vi "GetAlazar_SynthFocus_25.vi"(0 "AlazarCluster":T8, 1 "Digitizer Settings":T4={"Digitizer delay (us) "=0.0, "rf points per line"=2048, "lines per plane"=128, "Samp Rate (Hz)"=100000000.0, "Additional dig delay (us)"=0.0, "Voltage Scale"=0.4, "Pre-Looks"=0, "Offset delay (us)"=0.0, "bits A/D"=8, "Avg Num"=1, "DigTimeOut"=5.0, "Rel Dig Delay"=0.0, "Dig Ch"=0, "LeCroyCluster"={"LeCroy Channels"=[TRUE, FALSE, FALSE, FALSE], "LC read pt offset"=0.0, "Sweep Avg"=FALSE}, "Main Digitizer"=enum."NI Digitizer", "Dig Config"=enum."Single channel", "Digitizer ID Cluster"={"Acqiris/Alazar/SP ID"=[], "NI Instr Handles"=[], "LeCroy VISA"="", "GaGe Handle"={"Handle"=0, "Sample size"=0, "Resolution"=0, "Offset"=0, "Channels"=0, "Boards"=0}, "ATS Ref"="ATS9350", "Acqiris Address"=["PCI::INSTR0"], "ADQRef"=refnum, "adq_cu_ptr"=refnum}, "Trigger Settings"={"Trig Source"=1, "Trig Coupling"=0, "Trig Slope"=0, "Level (mV)"=1500.0}, "Bulk Acq"=FALSE, "Bulk Start Indexes"=[], "Data Ref RF"=refnum, "NI ID/Channel"=[], "Total Dig CH"=1, "Xtra Ann Trig delay (us)"=10.0, "Fix Z Delay?"=FALSE, "One Way Transmission?"=FALSE, "Data Ref Log"=refnum} {"Trigger Settings"."Trig Slope" items=["Positive", "Negative"]; "Trigger Settings"."Level (mV)" format="%.2f"; "Trigger Settings"."Trig Coupling" items=["DC 1 MOhm", "AC 1 MOhm", "DC 50 Ohm", "AC 50 Ohm"]; "Trigger Settings"."Trig Source" items=["Chan 1", "External"]; "Rel Dig Delay" format="%.2f"; "DigTimeOut" format="%.2f"; "Avg Num" min=1; "Offset delay (us)" format="%.2f"; "Additional dig delay (us)" format="%.2f"; "Digitizer delay (us)" format="%.2f"}, 7 "errorin":errorcluster, 8 "File Array":string[](array[string]), 9 "Ann Array Params":T1={"Synth Foc?"=FALSE, "Focal Zones"=41, "Switch T/R"=0, "Trans Geometry (mm)"={"Transducer"=0, "Geo Focus"=12.0, "a (radius)"=3.0, "# of rings"=5, "kerf space "=0.1, "Center Freq"=12.0}, "Sub Ap Excite?"=FALSE, "Full Array Scan?"=FALSE, "Xmt/Rcv"={"XMIT"=[TRUE, TRUE, TRUE, TRUE, TRUE], "RCV"=[TRUE, TRUE, TRUE, TRUE, TRUE]}, "PulseSpacing (us)"=0.0, "Xmit Ring"=0, "XMIT CHS"=0, "RCV CHS"=0, "GPU?"=FALSE, "Save TIFF?"=FALSE, "downfactor"=1, "RCV 1CH"=0} {"RCV 1CH" items=["All", "1", "2", "3", "4", "5"]; "Trans Geometry (mm)"."Transducer" items=["6D 12R 40 MHz"=0, "10D 31R 20 MHz"=1, "10D 23R 20 MHz"=2, "6D 23R 40 MHz"=3, "4.5D 10.7R 40 MHz"=4, "9D 23.5R 20 MHz"=5, "9D 25.8R 20MHz"=6, "Enter"=99]; "Switch T/R" min=1 max=5 step=1}, 10 "lines per plane":i32, 15 "Reverse?":bool) -> (17 "Raw VGain (scale)":dbl, 18 "Gain Array":T9(array[cluster]), 21 "VGain (dB)":dbl, 27 "error out":errorcluster)   [LabVIEW 2022 SP3]
uses:
  Motion Controllers/-MotionRoutines/MotionGlobals.vi
  Annular Array/-SynthApperture/ProcImageHD_I16.vi
  -DigitizerRoutines/DigitizerSettings.ctl
  -DigitizerRoutines/DigitizerID.ctl
  -DigitizerRoutines/Digitizer.ctl
  Annular Array/-AnnularRoutines/ArrayGeometry.ctl
  Annular Array/-AnnularRoutines/TransGeometry.ctl
  Annular Array/-AnnularRoutines/AnnularArray.ctl
  -DigitizerRoutines/DigConfig.ctl
  C:/Windows/System32/ADQAPI_dotNet_helper.dll
panel:
  out "read time":u32
  out "save time":u32
  out "Numeric":i32
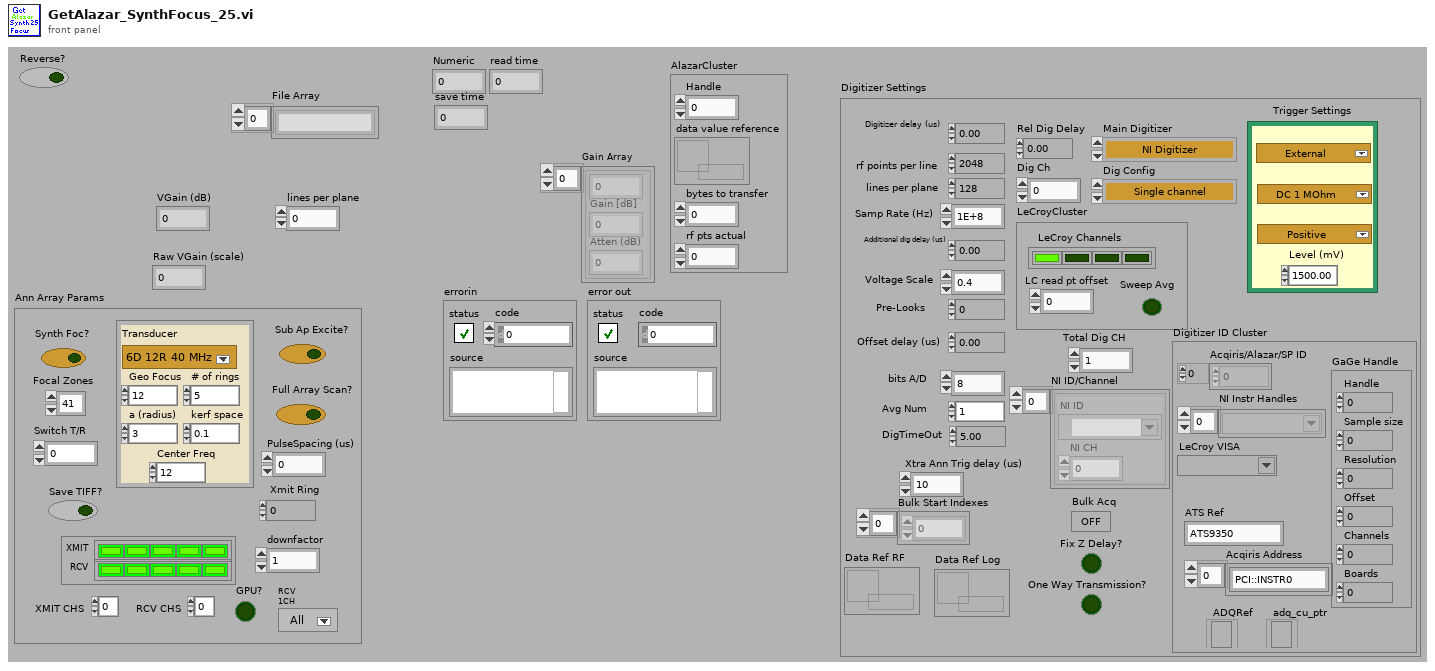
[diagram p1: front panel]
types:
  T1 = typedef "AnnularArray.ctl" = cluster{"Synth Foc?":bool, "Focal Zones":i16, "Switch T/R":i16, "Trans Geometry (mm)":T2, "Sub Ap Excite?":bool, "Full Array Scan?":bool, "Xmt/Rcv":cluster{"XMIT":bool[], "RCV":bool[]}, "PulseSpacing (us)":sgl, "Xmit Ring":i32, "XMIT CHS":u8, "RCV CHS":u8, "GPU?":bool, "Save TIFF?":bool, "downfactor":i32, "RCV 1CH":u16}
  T2 = typedef "TransGeometry.ctl" = cluster{"Transducer":T3, "Geo Focus":dbl, "a (radius)":dbl, "# of rings":i32, "kerf space ":dbl, "Center Freq":dbl}
  T3 = typedef "ArrayGeometry.ctl" = u16
  T4 = typedef "DigitizerSettings.ctl" = cluster{"Digitizer delay (us) ":dbl, "rf points per line":i32, "lines per plane":i32, "Samp Rate (Hz)":dbl, "Additional dig delay (us)":dbl, "Voltage Scale":dbl, "Pre-Looks":i32, "Offset delay (us)":dbl, "bits A/D":i8, "Avg Num":i32, "DigTimeOut":sgl, "Rel Dig Delay":sgl, "Dig Ch":i32, "LeCroyCluster":cluster{"LeCroy Channels":bool[], "LC read pt offset":dbl, "Sweep Avg":bool}, "Main Digitizer":T5, "Dig Config":T6, "Digitizer ID Cluster":T7, "Trigger Settings":cluster{"Trig Source":u16, "Trig Coupling":u16, "Trig Slope":u16, "Level (mV)":dbl}, "Bulk Acq":bool, "Bulk Start Indexes":i32[], "Data Ref RF":refnum<data-value>, "NI ID/Channel":cluster{"NI ID":refnum<k15>, "NI CH":i32}[], "Total Dig CH":i32, "Xtra Ann Trig delay (us)":dbl, "Fix Z Delay?":bool, "One Way Transmission?":bool, "Data Ref Log":refnum<data-value>}
  T5 = typedef "Digitizer.ctl" = enum16{"Acqiris Digitizer", "NI Digitizer", "LeCroy", "GaGe", "AlazarTech", "No Digitizer", "Teledyne"}
  T6 = typedef "DigConfig.ctl" = enum16{"Single channel", "2 Chans w/ 2 Acqiris", "2 Chans w/ 1 Acqiris", "5-CH Pulser New", "5-CH pulser w/ ann array", "5-pass style ann array", "Empty"}
  T7 = typedef "DigitizerID.ctl" = cluster{"Acqiris/Alazar/SP ID":u32[], "NI Instr Handles":refnum<k15>[], "LeCroy VISA":refnum<visa-resource-name>, "GaGe Handle":cluster{"Handle":u32, "Sample size":u32, "Resolution":i32, "Offset":i32, "Channels":u32, "Boards":u32}, "ATS Ref":string, "Acqiris Address":string[], "ADQRef":refnum<k24>, "adq_cu_ptr":refnum<k24>}
  T8 = cluster{"Handle":u32, "data value reference":refnum<data-value>, "bytes to transfer":u32, "rf pts actual":u32}
  T9 = cluster{sgl, "Gain [dB]  ":sgl, "Atten (dB)":sgl}[]
  T10 = cluster{"wfm":i16[][], "max queue size (-1, unlimited)":i32}
  T11 = cluster{sgl, "Gain [dB]  ":sgl, "Atten (dB)":sgl}
  T12 = cluster{"low cutoff":i32, "order":i32, "high cutoff":i32}
  T13 = cluster{"FIR Windowed Coefficients":dbl[], "Filter Prams":cluster{"low cutoff":i32, "order":i32, "high cutoff":i32}}
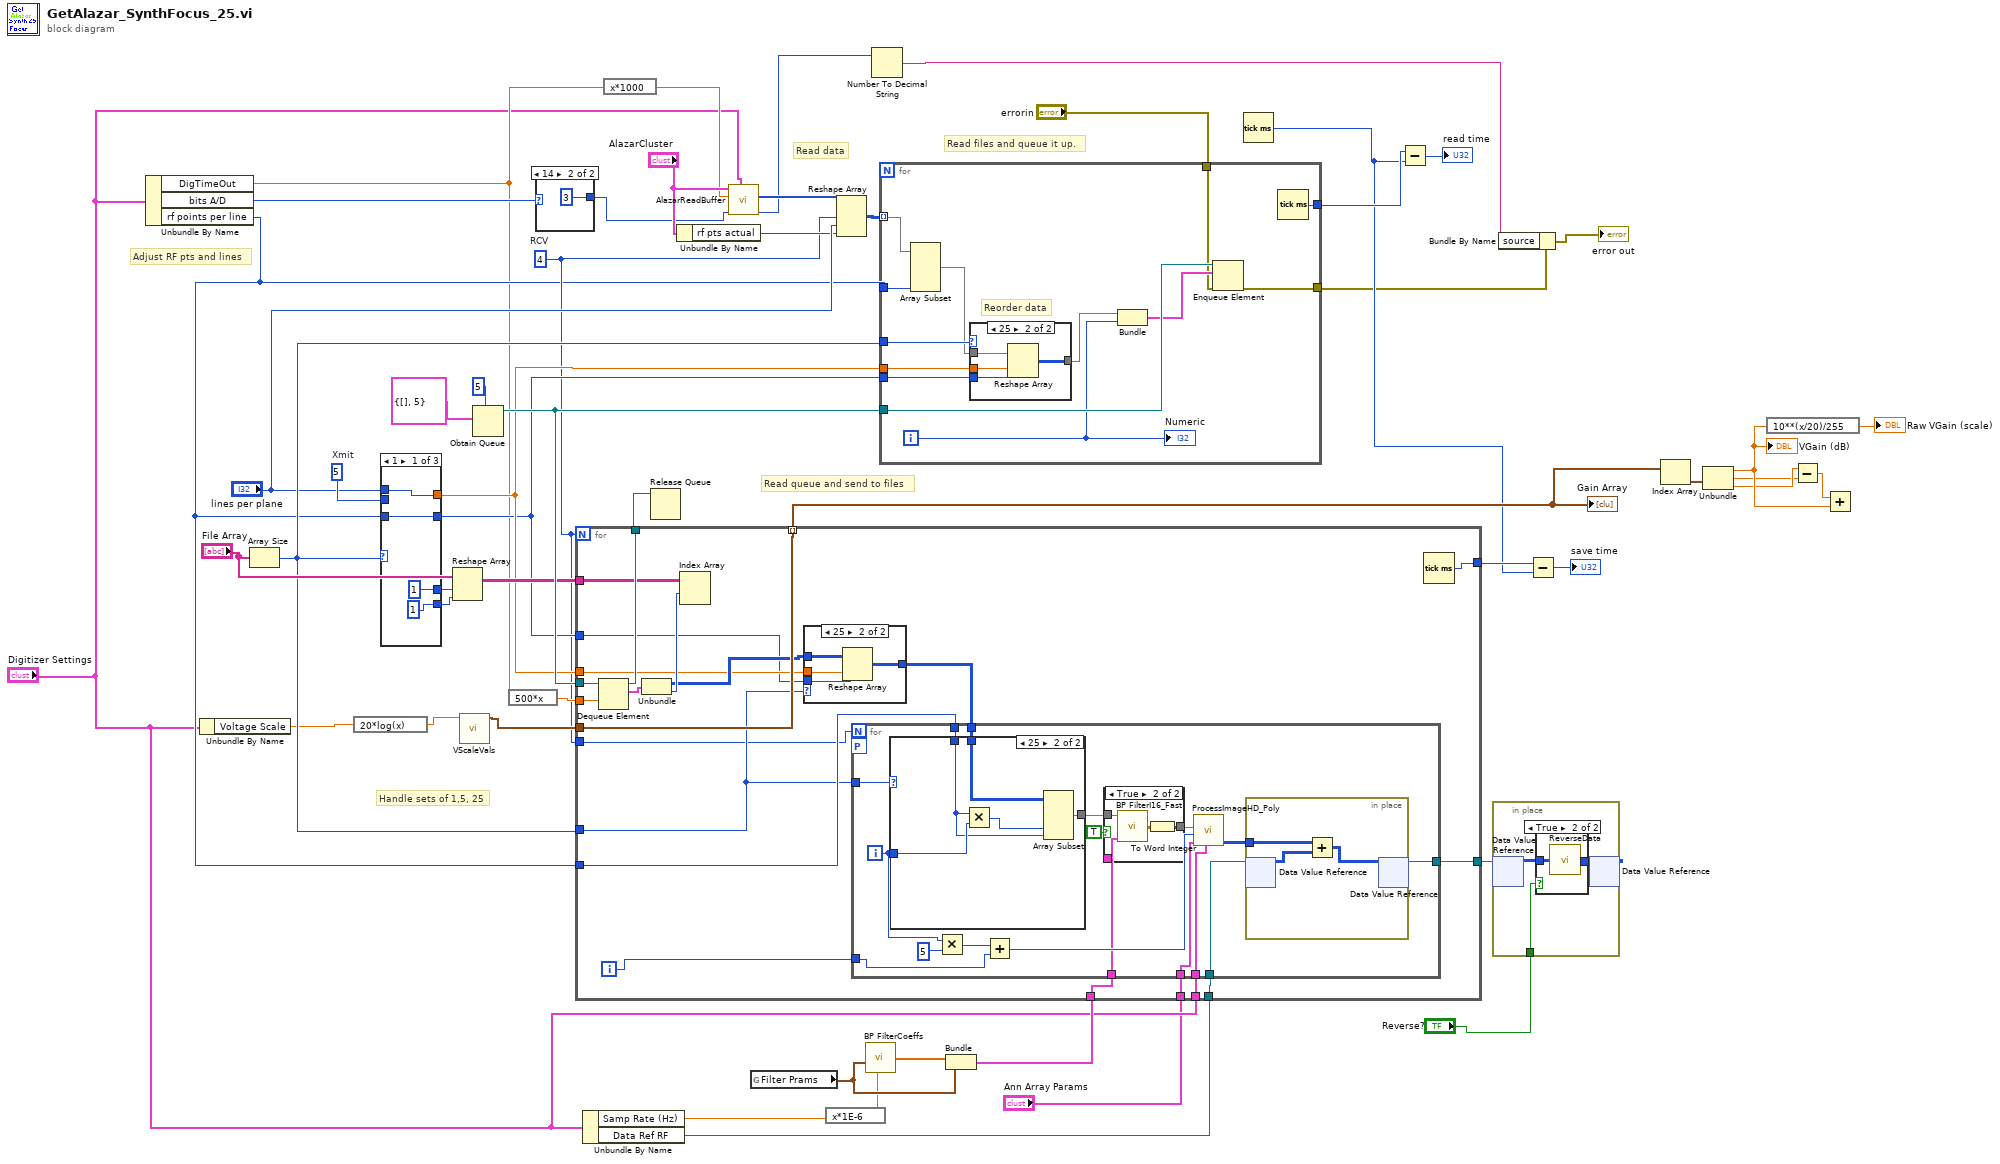
[diagram p0: block diagram]
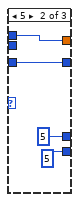
[diagram p5: hidden frame]
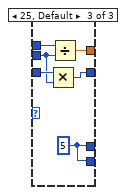
[diagram p6: hidden frame]
diagram:
  w30 = 5  # Xmit
  w11 = 4  # RCV
  # "Read data"
  # "Adjust RF pts and lines"
  # "Handle sets of 1,5, 25"
  # "Read files and queue it up."
  # "Read queue and send to files"
  n1 = Unbundle By Name("Digitizer Settings") -> ("DigTimeOut"=w6:sgl, "bits A/D"=w7:i8, "rf points per line"=w8:i32)
  n2 = Unbundle By Name("Digitizer Settings") -> ("Voltage Scale"=w10:dbl)
  n3 = Array Size(array="File Array") -> (size(s)=w34:i32)
  n4 = expression code="20*log(x)"(w10) -> (w32:dbl)
  n5 = case shown="1" w34 {
    tunnel: [1 5 w68] -> w37
    tunnel: [w57 w61 w64] -> w16
    tunnel: w8 -> [w57 w61 w65]
    tunnel: [w56 w60 w66] -> w17
    tunnel: "lines per plane" -> [w56 w60 w67]
    tunnel: [1 5 w68] -> w36
    tunnel: w30 -> [_ _ w63]
    frame 1 {
    }
    frame 5 {
    }
    frame 25, Default {
      w68 = 5
      n6 = Multiply(x=w65, y=w63) -> (x*y=w64:i32)
      n7 = Divide(x=w67, y=w63) -> (x/y=w66:dbl)
    }
  }
  n8 = Reshape Array("File Array", w37, w36) -> (w33:string[][])
  n9 = call "VScaleVals.vi"("Full Scale"=w32) -> ("Voltage Scale"=w31:T11)  [unwired: 8 in, 2 out]
  n10 = Obtain Queue(max queue size (-1, unlimited)=5, element data type=T10 {"wfm"=[], "max queue size (-1, unlimited)"=5}) -> (queue out=w46:refnum<queue>)  [unwired: 3 in, 2 out]
  n11 = expression code="500*x"(w6) -> (w35:sgl)
  n12 = case shown="14" w7 {
    tunnel: [_ u16 3 ("Extra Shift")] -> w18
    frame 0, Default {
    }
    frame 14 {
    }
  }
  n13 = Unbundle By Name("Digitizer Settings") -> ("Samp Rate (Hz)"=w9:dbl, "Data Ref RF"=w4:refnum<data-value>)
  n14 = expression code="x*1000"(w6) -> (w23:sgl)
  n15 = Unbundle By Name("AlazarCluster") -> ("rf pts actual"=w26:u32)
  n16 = call "AlazarReadBuffer.vi"("Digitizer Settings"="Digitizer Settings", "Extra Shift"=w18, "time out"=w23, "AlazarCluster"="AlazarCluster") -> ("Return Code"=w19:u32, "Data Array"=w27:i16[])  [unwired: 5 in, 1 out]
  n17 = global read "MotionGlobals.vi" "Filter Prams"() -> (w15:T12)
  n18 = expression code="x*1E-6"(w9) -> (w14:dbl)
  n19 = Reshape Array(w27, w11, "lines per plane", w26) -> (w25:i16[][][])
  n20 = call "BP FilterCoeffs.vi"("sample rate MHz"=w14, "Filter Prams"=w15) -> ("FIR Windowed Coefficients"=w13:dbl[])  [unwired: 4 in]
  n21 = Number To Decimal String(number=w19) -> (decimal integer string=w21:string)  [unwired: 1 in]
  n22 = for {
    tunnel: w46 -> [w82]
    tunnel: [w80] -> w44
    tunnel: [w79] -> w22
    tunnel: w34 -> [w78]
    tunnel: w17 -> [w77]
    tunnel: w16 -> [w76]
    tunnel: w25 -> [w74] mode=indexing
    tunnel: w8 -> [w73]
    tunnel: "errorin" -> [w70]
    i -> [w71]
    # "Reorder data"
    n23 = Array Subset(array=w74, length (col)=w73) -> (w72:i16[][])  [unwired: 3 in]
    n24 = case shown="25" w78 {
      tunnel: w76 -> [_ w87]
      tunnel: w72 -> [w83 w86]
      tunnel: [w83 w85] -> w75
      tunnel: w77 -> [_ w84]
      frame 0, Default {
      }
      frame 25 {
        n25 = Reshape Array(w86, w84, w87) -> (w85:i16[][])
      }
    }
    n26 = Bundle(w75, w71) -> (w81:cluster{i16[][], i32})  [unwired: 1 in]
    n27 = Enqueue Element(queue=w82, element=w81, error in (no error)=w70) -> (error out=w79:errorcluster)  [unwired: 1 in, 2 out]
    n28 = Tick Count (ms)() -> (millisecond timer value=w80:u32)
    "Numeric" <- w71
  }
  n29 = Bundle("FIR Windowed Coefficients"=w13, "Filter Prams"=w15) -> (w12:T13)  [unwired: 1 in]
  n30 = for {
    N: w11 -> [_]
    tunnel: w8 -> [w96]
    tunnel: [w102] -> w47 mode=indexing
    tunnel: w46 -> [w108]
    tunnel: [w106] -> w39
    tunnel: [w105] -> w43
    tunnel: w34 -> [w95]
    tunnel: w35 -> [w104]
    tunnel: w33 -> [w103]
    tunnel: w31 -> [w102]
    tunnel: w17 -> [w99]
    tunnel: w16 -> [w98]
    tunnel: w12 -> [w94]
    tunnel: w4 -> [w93]
    tunnel: w11 -> [w91]
    tunnel: "Digitizer Settings" -> [w90]
    tunnel: "Ann Array Params" -> [w89]
    tunnel: [w88] -> w2
    i -> [w92]
    n31 = Dequeue Element(queue=w108, timeout in ms (-1)=w104) -> (queue out=w106:refnum<queue>, element=w107:T10)  [unwired: 1 in, 2 out]
    n32 = Unbundle(w107) -> ("wfm"=w100:i16[][], "max queue size (-1, unlimited)"=w101:i32)
    n33 = Index Array(array=w103, index (row)=w101) -> ()  [unwired: 1 in, 1 out]
    n34 = case shown="25" w95 {
      tunnel: w98 -> [_ w144]
      tunnel: w100 -> [w140 w143]
      tunnel: [w140 w142] -> w97
      tunnel: w99 -> [_ w141]
      frame 0, Default {
      }
      frame 25 {
        n35 = Reshape Array(w143, w141, w144) -> (w142:i16[][])
      }
    }
    n36 = for {
      N: w91 -> [_]
      tunnel: w96 -> [w125]
      tunnel: w97 -> [w124]
      workers-P: _ -> [_]
      tunnel: w95 -> [w123]
      tunnel: w93 -> [w117]
      tunnel: w94 -> [w114]
      tunnel: w92 -> [w112]
      tunnel: w90 -> [w111]
      tunnel: w89 -> [w110]
      tunnel: [w109] -> w88
      i -> [w122]
      n37 = case shown="25" w123 {
        tunnel: [w134 w135] -> w116
        tunnel: w122 -> [_ w139]
        tunnel: w125 -> [_ w137]
        tunnel: w124 -> [w134 w136]
        frame 5, Default {
        }
        frame 25 {
          n38 = Multiply(x=w137, y=w139) -> (x*y=w138:i32)
          n39 = Array Subset(array=w136, index (col)=w138, length (col)=w137) -> (w135:i16[][])  [unwired: 2 in]
        }
      }
      n40 = Multiply(x=w122, y=5 ("max queue size (-1, unlimited)")) -> (x*y=w120:i32)
      n41 = Add(x=w120, y=w112) -> (x+y=w119:i32)
      n42 = case shown="True" TRUE {
        tunnel: w116 -> [w126 w129]
        tunnel: [w126 w128] -> w115
        tunnel: w114 -> [_ w127]
        frame False {
        }
        frame True {
          n43 = call "BP FilterI16_Fast.vi"("Filter"=w127, "Array in"=w129) -> ("Filtered X"=w130:dbl[][])  [unwired: 4 in]
          n44 = To Word Integer(number=w130) -> (16bit integer=w128:i16[][])
        }
      }
      n45 = call-poly "ProcessImageHD_Poly.vi"("Digitizer Settings"=w111, "Ann Array Params"=w110, "T/R Ring"=w119, "Scan Data In"=w115) -> ("Synth App Out"=w118:i16[][])  [unwired: 4 in, 1 out]
      n46 = in-place {
        in-place-border: w118 -> [w131]
        n47 = in-place-dvr #1(w117) -> (w133:i16[][])  [unwired: 1 out]
        n48 = Add(x=w131, y=w133) -> (x+y=w132:i16[][])
        n49 = in-place-dvr #1(w132) -> (w109:refnum<data-value>)  [unwired: 1 out]
      }
    }
    n50 = Tick Count (ms)() -> (millisecond timer value=w105:u32)
  }
  "Gain Array" <- w47
  n51 = Release Queue(queue=w39) -> ()  [unwired: 2 in, 3 out]
  n52 = Tick Count (ms)() -> (millisecond timer value=w42:u32)
  n53 = Subtract(x=w44, y=w42) -> (x-y=→"read time":u32)
  n54 = in-place {
    in-place-border: "Reverse?" -> [w145]
    n55 = in-place-dvr #2(w2) -> (w147:i16[][])  [unwired: 1 out]
    n56 = case shown="True" w145 {
      tunnel: w147 -> [w148 w150]
      tunnel: [w148 w149] -> w146
      frame False {
      }
      frame True {
        n57 = call "ReverseData.vi"("Array in"=w150) -> ("Array out"=w149:i16[][])
      }
    }
    n58 = in-place-dvr #2(w146) -> ()  [unwired: 2 out]
  }
  n59 = Bundle By Name(cluster=w22, "source"=w21) -> (→"error out":errorcluster)
  n60 = Subtract(x=w43, y=w42) -> (x-y=→"save time":u32)
  n61 = Index Array(array=w47) -> (element=w54:T11)  [unwired: 1 in]
  n62 = Unbundle(w54) -> (w53:sgl, "Gain [dB]"=w51:sgl, "Atten (dB)"=w52:sgl)
  "VGain (dB)" <- w53
  n63 = expression code="10**(x/20)/255"(w53) -> (→"Raw VGain (scale)":sgl)
  n64 = Subtract(x=w52, y=w51) -> (x-y=w50:sgl)
  n65 = Add(x=w50, y=w53) -> ()  [unwired: 1 out]
